vi "Query Int.vi"(8 "error in (no error)":errorcluster, 10 "write buffer":string, 11 "VISA resource name In":refnum<visa-resource-name>) -> (0 "error out":errorcluster, 2 "int":u32, 3 "VISA resource name out":refnum<visa-resource-name>)   [LabVIEW 2012, in "Newport 1830-C.lvlib"]
doc: "Reads the and unsigned 32-bit integer from the output buffer of the instrument."
uses:
  Newport 1830-C.lvlib
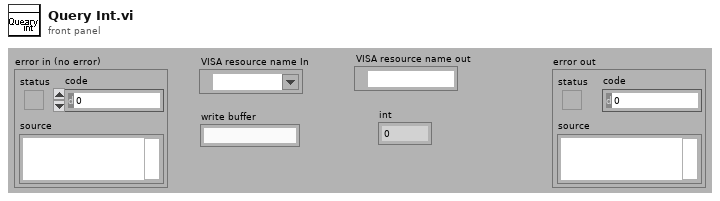
[diagram p1: front panel]
types:
  T1 = typedef "Semaphore RefNum" = refnum<k1>
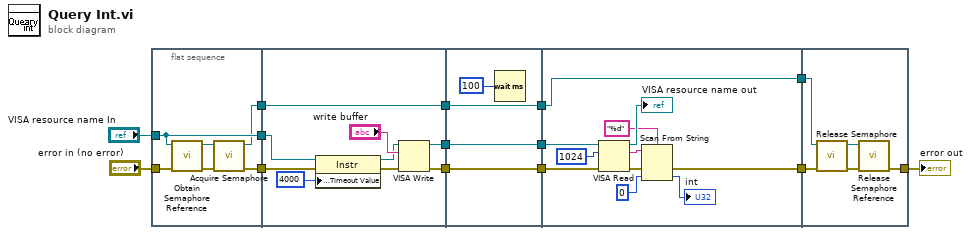
[diagram p0: block diagram]
diagram:
  n1 = flat-sequence {
    tunnel: "error in (no error)" -> [w20]
    tunnel: "VISA resource name In" -> [w16]
    tunnel: [w17] -> w12
    tunnel: [w16] -> w11
    tunnel: [w15] -> w1
    tunnel: w12 -> [w24]
    tunnel: w11 -> [w25]
    tunnel: [w28] -> w9
    tunnel: [w27] -> w7
    tunnel: [w26] -> w2
    tunnel: w1 -> [w26]
    tunnel: [w32] -> w10
    tunnel: w9 -> [w32]
    tunnel: [w31] -> w8
    tunnel: w7 -> [w31]
    tunnel: [w30] -> w3
    tunnel: w2 -> [w30]
    tunnel: w10 -> [w37]
    tunnel: w8 -> [w36]
    tunnel: [w35] -> w6
    tunnel: [w34] -> w4
    tunnel: w3 -> [w34]
    tunnel: w6 -> [w49]
    tunnel: [w47] -> w5
    tunnel: w4 -> [w46]
    frame #0 {
      n2 = call <vilib>:"Obtain Semaphore Reference.vi"("error in (no error)"=w20, "name (unnamed)"=w16) -> ("error out"=w18:errorcluster, "semaphore"=w19:T1)  [unwired: 3 in, 1 out]
      n3 = call <vilib>:"Acquire Semaphore.vi"("error in (no error)"=w18, "semaphore"=w19) -> ("error out"=w17:errorcluster, "semaphore out"=w15:T1)  [unwired: 3 in, 1 out]
    }
    frame #1 {
      n4 = property class="Instr"(reference=w25, error in=w24, "General Settings:Timeout Value"=u32 4000) -> (reference out=w22:refnum<visa-resource-name>, error out=w23:errorcluster)
      n5 = VISA Write(VISA resource name=w22, write buffer="write buffer", error in (no error)=w23) -> (VISA resource name out=w27:refnum<visa-resource-name>, error out=w28:errorcluster)  [unwired: 1 out]
    }
    frame #2 {
      n6 = Wait (ms)(milliseconds to wait=u32 100) -> ()  [unwired: 1 out]
    }
    frame #3 {
      n7 = VISA Read(VISA resource name=w36, byte count=u32 1024, error in (no error)=w37) -> (VISA resource name out=→"VISA resource name out":refnum<visa-resource-name>, read buffer=w39:string, error out=w40:errorcluster)  [unwired: 1 out]
      n8 = Scan From String(format string="%d", input string=w39, error in=w40, default 1=u32 0) -> (error out=w35:errorcluster, output 1=→"int":u32)  [unwired: 1 in, 2 out]
    }
    frame #4 {
      n9 = call <vilib>:"Release Semaphore.vi"("error in (no error)"=w49, "semaphore"=w46) -> ("error out"=w48:errorcluster, "semaphore out"=w45:T1)  [unwired: 4 in]
      n10 = call <vilib>:"Release Semaphore Reference.vi"("error in (no error)"=w48, "semaphore"=w45) -> ("error out"=w47:errorcluster)  [unwired: 8 in, 1 out]
    }
  }
  "error out" <- w5
